vi "Add Master Queue.vi"(8 "error in (no error)":errorcluster, 10 "Master Actor Q":refnum<class "Message Enqueuer.lvclass">, 11 "DAQ Actor (Slave)":refnum<class "DAQ Actor (Slave).lvclass">) -> (0 "error out":errorcluster, 3 "DAQ Actor (Slave) out":refnum<class "DAQ Actor (Slave).lvclass">)   [LabVIEW 2018, in "Data Acquisition.lvlib" / "DAQ Actor (Slave).lvclass"]
uses:
  DAQ Actor (Slave).lvclass
  <vilib>/ActorFramework/Message Enqueuer/Message Enqueuer.lvclass
  DAQ Actor (Slave).lvclass/DAQ Actor (Slave).ctl
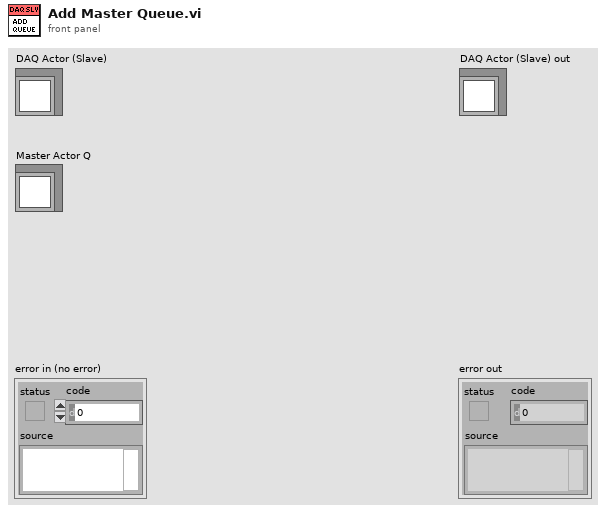
[diagram p1: front panel]
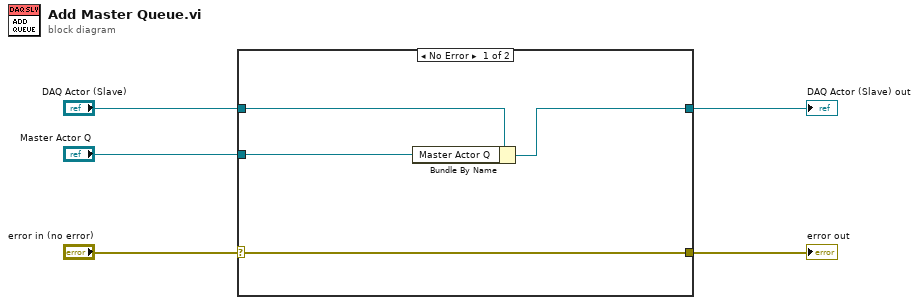
[diagram p0: block diagram]
diagram:
  n1 = case shown="No Error" "error in (no error)" {
    selector: "error in (no error)" -> [w9 w11]
    tunnel: [w9 w11] -> w5
    tunnel: [w7 w10] -> w4
    tunnel: "DAQ Actor (Slave)" -> [w8 w10]
    tunnel: "Master Actor Q" -> [w6 _]
    frame No Error {
      n2 = Bundle By Name(cluster=w8, "Master Actor Q"=w6) -> (w7:refnum<class "DAQ Actor (Slave).lvclass">)
    }
    frame Error {
    }
  }
  "error out" <- w5
  "DAQ Actor (Slave) out" <- w4
